vi "Arm Controls.vi"(11 "Robot Commands":T1) -> ()   [LabVIEW 2015]
uses:
  Joystick/Robot Commands.ctl
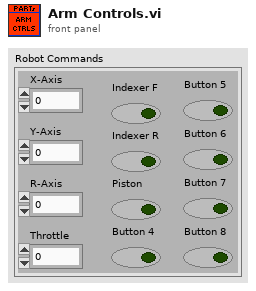
[diagram p1: front panel]
types:
  T1 = typedef "Robot Commands.ctl" = cluster{"X-Axis":dbl, "Y-Axis":dbl, "R-Axis":dbl, "Throttle":dbl, "Indexer F":bool, "Indexer R":bool, "Piston":bool, "Button 4":bool, "Button 5":bool, "Button 6":bool, "Button 7":bool, "Button 8":bool}
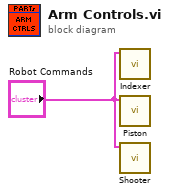
[diagram p0: block diagram]
diagram:
  n1 = call "Indexer.vi"("Robot Commands"="Robot Commands") -> ()  [unwired: 11 in]
  n2 = call "Piston.vi"("Robot Commands"="Robot Commands") -> ()  [unwired: 11 in]
  n3 = call "Shooter.vi"("Robot Commands"="Robot Commands") -> ()  [unwired: 11 in]
